vi "Get All Logger Info.vi"(8 "error in":errorcluster) -> (0 "error out":errorcluster, 3 "logger info":T2(array[cluster]))   [LabVIEW 2018, in "GLog.lvlib"]
uses:
  GLog.lvlib
  Log Levels.ctl
  registry/Registry.lvlib
panel:
  # "Connector Pane"
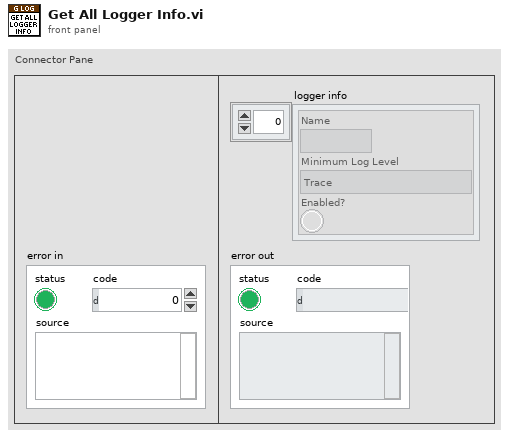
[diagram p1: front panel]
types:
  T1 = typedef "GLog.lvlib/Log Levels.ctl" = enum16{"Trace", "Debug", "Info", "Warning", "Error", "Critical"}
  T2 = cluster{"Name":string, "Minimum Log Level":T1, "Enabled?":bool}[]
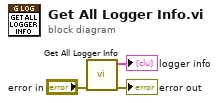
[diagram p0: block diagram]
diagram:
  n1 = call "Get All Logger Info.vi"("error in"="error in") -> ("error out"=→"error out":errorcluster, "logger info"=→"logger info":T2)  [unwired: 9 in]
